vi "等高线.vi"() -> ()   [LabVIEW 2012]
uses:
  <vilib>/Math Plots/3D Math Plots/3D Contour/3D Contour XCtrl/3D Contour.xctl
  <vilib>/imath/engines/lvmath/Plug In/_Char/NIMS_CH_character datatype.ctl
  <vilib>/Math Plots/3D Math Plots/3D Contour/3D Contour Datatype/Public/Plot Helper (Matrix).vi
  <vilib>/imath/engines/lvmath2/RunTimeEngine/ErrorHandling/NIMS_Finalize Error.vi
  <vilib>/imath/engines/lvmath2/RunTimeEngine/NodeEndStatement/NIMS_NodeEndStatement_Output.vi
  <instcachedir>/0/NIMS_NodeEndStatement_Output_53EC0D466D134D7ABD903AC30B43404B.lvgen/NIMS_NodeEndStatement_Output_53EC0D466D134D7ABD903AC30B43404B_002.vi
  <vilib>/imath/engines/lvmath2/RunTimeEngine/BuiltInFunctions/peakfcn2d/NIMS_peakfcn2d(I32S).vi
  <vilib>/imath/engines/lvmath2/RunTimeEngine/ErrorHandling/NIMS_Error From Error Code.vi
  <vilib>/imath/engines/lvmath2/RunTimeEngine/BuiltInFunctions/contour/NIMS_contour(M, M, S).vi
  <vilib>/imathl/engines/lvmath/Functions/Error Handling/Create Error.vi
  <vilib>/imath/engines/lvmath/Plug In/_Char/NIMS_CH_Character RV to String.vi
  <vilib>/imath/engines/lvmath2/RunTimeEngine/BuiltInFunctions/title/NIMS_title.vi
  <vilib>/imath/engines/lvmath2/RunTimeEngine/BuiltInFunctions/pause/NIMS_pause(S).vi
  <vilib>/imath/engines/lvmath2/RunTimeEngine/BuiltInFunctions/contouris/NIMS_contouris(M, M, S).vi
  <vilib>/imath/engines/lvmath2/RunTimeEngine/BuiltInFunctions/contour3d/NIMS_contour3d(M, M, S).vi
  <vilib>/Math Plots/3D Math Plots/3D Contour/3D Contour Datatype/3D Contour Datatype.lvclass
panel:
  out "3D Contour":refnum<class "3D Plot Datatype.lvclass">[](xcontrol) caption="三维等高线"
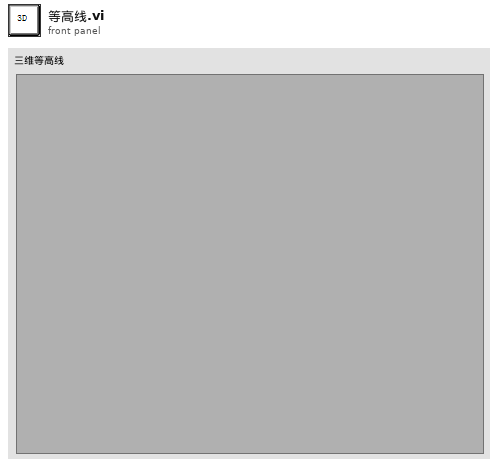
[diagram p1: front panel]
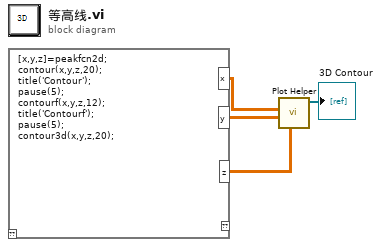
[diagram p0: block diagram]
diagram:
  n1 = mathscript code="[x,y,z]=peakfcn2d;\ncontour(x,y,z,20);\ntitle('Contour');\npause(5);\ncontourf(x,y,z,12);\ntitle('Contourf');\npause(5);\ncontour3d(x,y,z,20);"() -> ("x"=w3:dbl[][], "y"=w2:dbl[][], "z"=w1:dbl[][])  [unwired: 1 in, 1 out]
  n2 = call-poly <vilib>:"Plot Helper.vi"("z matrix"=w1, "y matrix"=w2, "x matrix"=w3) -> ("3D Plot lvclass Array out"=→"3D Contour":refnum<class "3D Plot Datatype.lvclass">[])  [unwired: 3 in, 5 out]
